vi "Paint Path.vi"(6 "color(Green)":u32(colorbox)=6618880, 8 "Starting Pos":cluster{"x":i16, "y":i16}, 9 "new picture in":picture, 10 "Array":string[](array[string]), 11 "Digital in":refnum<vi>) -> (3 "new picture out":picture)   [LabVIEW 2018]
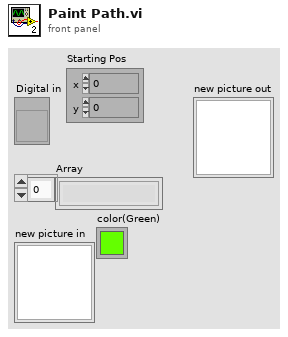
[diagram p1: front panel]
types:
  T1 = cluster{"Width":u16, "Style":enum32{"Solid", "Dash", "Dot", "DashDot", "DashDotDot"}}
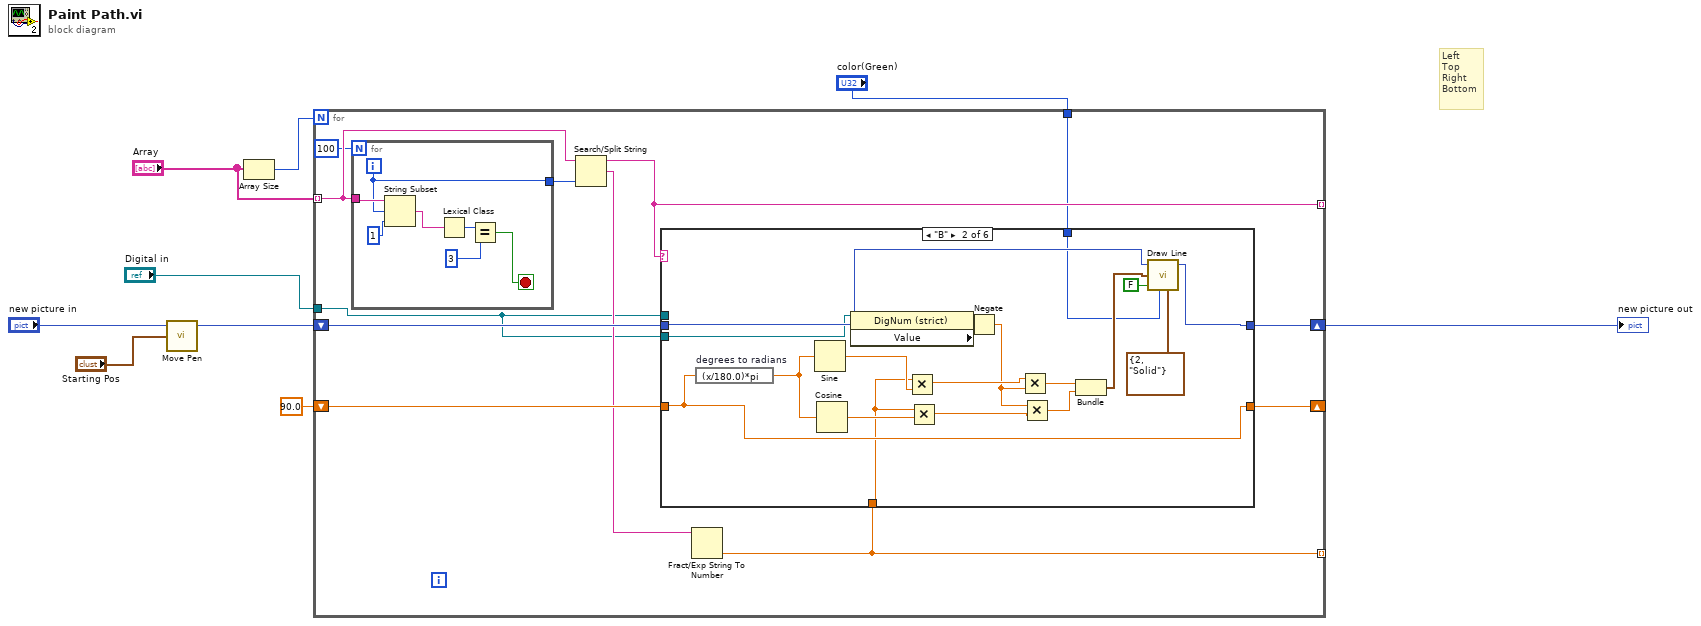
[diagram p0: block diagram]
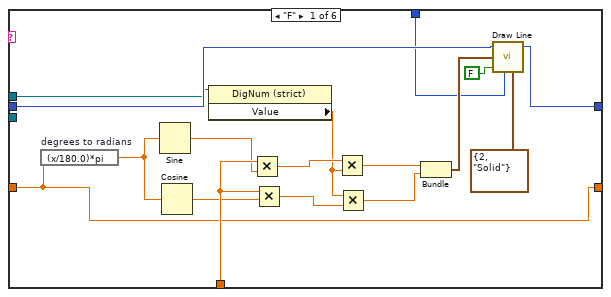
[diagram p2: hidden frame]
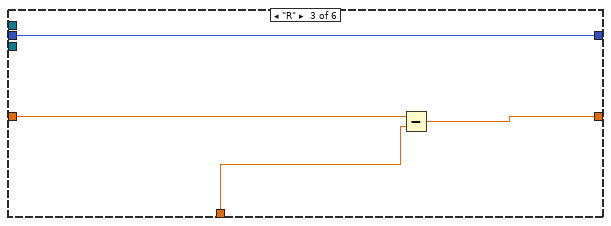
[diagram p3: hidden frame]
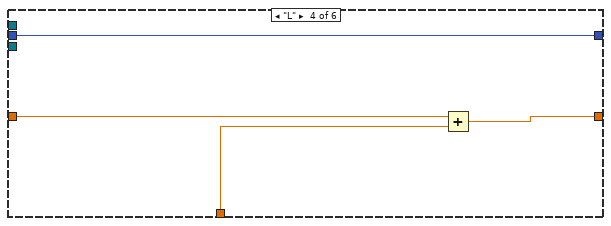
[diagram p4: hidden frame]
diagram:
  # "Left\nTop\nRight\nBottom"
  n1 = call <vilib>:"Move Pen.vi"("new position"="Starting Pos", "picture"="new picture in") -> ("new picture"=w3:picture)  [unwired: 3 in]
  n2 = Array Size(array="Array") -> (size(s)=w9:i32)
  n3 = for {
    N: w9 -> [_]
    tunnel: [w21] -> _ mode=indexing
    tunnel: [w14] -> _ mode=indexing
    tunnel: "Array" -> [w15] mode=indexing
    shift-right: [w19] -> w7
    shift-left: w3 -> [w20]
    shift-right: [w17] -> _
    shift-left: 90.0 -> [w18]
    tunnel: "Digital in" -> [w11]
    tunnel: "color(Green)" -> [w10]
    n4 = for {
      N: 100 -> [_]
      tunnel: w15 -> [w73]
      tunnel: [w70] -> w16
      i -> [w70]
      stop <- w69 stop-if-true
      n5 = String Subset(string=w73, offset (0)=w70, length (rest)=1 ("length (rest)")) -> (substring=w71:string)
      n6 = Lexical Class(1:w71) -> (0:w75:i16)
      n7 = Equal?(x=w75, y=i16 3) -> (x = y?=w69:bool)
    }
    n8 = Search/Split String(string=w15, offset (0)=w16) -> (substring before match=w14:string, match + rest of string=w13:string)  [unwired: 1 in, 1 out]
    n9 = Fract/Exp String To Number(string=w13) -> (number=w21:dbl)  [unwired: 3 in, 1 out]
    n10 = case shown="\"B\"" w14 {
      tunnel: w21 -> [w35 w48 w57 w61 _ _]
      tunnel: w20 -> [w37 w51 w60 w64 w66 w68]
      tunnel: [w36 w50 w60 w64 w66 w68] -> w19
      tunnel: w18 -> [w31 w49 w58 w62 w65 w67]
      tunnel: [w31 w49 w59 w63 w65 w67] -> w17
      tunnel: w11 -> [w23 _ _ _ _ _]
      tunnel: w11 -> [_ w40 _ _ _ _]
      tunnel: w10 -> [w22 w39 _ _ _ _]
      frame "F" {
        n11 = expression code="(x/180.0)*pi" "degrees to radians"(w31) -> (w34:dbl)
        n12 = Sine(x=w34) -> (sin(x)=w32:dbl)
        n13 = Cosine(x=w34) -> (cos(x)=w33:dbl)
        n14 = property class="DigNum (strict)"(reference=w23) -> ("Value"=w24:dbl)  [unwired: 1 in, 2 out]
        n15 = Multiply(x=w35, y=w32) -> (x*y=w27:dbl)
        n16 = Multiply(x=w35, y=w33) -> (x*y=w28:dbl)
        n17 = Multiply(x=w27, y=w24) -> (x*y=w26:dbl)
        n18 = Multiply(x=w24, y=w28) -> (x*y=w25:dbl)
        n19 = Bundle(w26, w25) -> (w29:cluster{dbl, dbl})  [unwired: 1 in]
        n20 = call <vilib>:"Draw Line.vi"("picture"=w37, "end point"=w29, "absolute coordinates?(T)"=FALSE, "color(black)"=w22, "pen"=T1 {"Width"=2, "Style"=enum."Solid"}) -> ("new picture"=w36:picture)  [unwired: 4 in]
      }
      frame "B" {
        n21 = expression code="(x/180.0)*pi" "degrees to radians"(w49) -> (w54:dbl)
        n22 = Sine(x=w54) -> (sin(x)=w52:dbl)
        n23 = Cosine(x=w54) -> (cos(x)=w53:dbl)
        n24 = property class="DigNum (strict)"(reference=w40) -> ("Value"=w46:dbl)  [unwired: 1 in, 2 out]
        n25 = Multiply(x=w48, y=w52) -> (x*y=w44:dbl)
        n26 = Multiply(x=w48, y=w53) -> (x*y=w45:dbl)
        n27 = Negate(x=w46) -> (-x=w41:dbl)
        n28 = Multiply(x=w44, y=w41) -> (x*y=w43:dbl)
        n29 = Multiply(x=w41, y=w45) -> (x*y=w42:dbl)
        n30 = Bundle(w43, w42) -> (w55:cluster{dbl, dbl})  [unwired: 1 in]
        n31 = call <vilib>:"Draw Line.vi"("picture"=w51, "end point"=w55, "absolute coordinates?(T)"=FALSE, "color(black)"=w39, "pen"=T1 {"Width"=2, "Style"=enum."Solid"}) -> ("new picture"=w50:picture)  [unwired: 4 in]
      }
      frame "R" {
        n32 = Subtract(x=w58, y=w57) -> (x-y=w59:dbl)
      }
      frame "L" {
        n33 = Add(x=w62, y=w61) -> (x+y=w63:dbl)
      }
      frame "D", Default {
      }
      frame "IF" {
      }
    }
  }
  "new picture out" <- w7
